vi "init_electron_count_Q.vi"(2 "max queue size (-1, unlimited)":i32) -> (8 "Electron Count Q Out":T1)   [LabVIEW 2023]
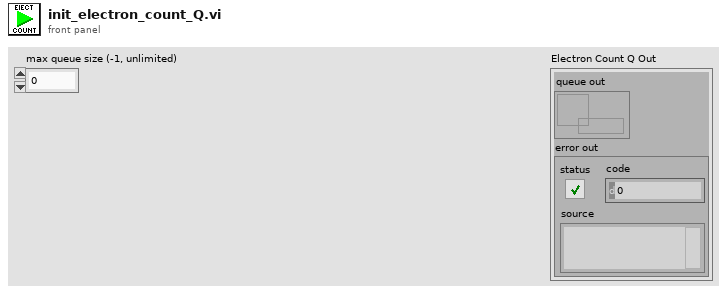
[diagram p1: front panel]
types:
  T1 = cluster{"queue out":refnum<queue>, "error out":errorcluster}
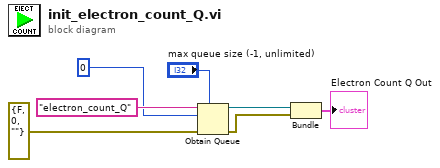
[diagram p0: block diagram]
diagram:
  n1 = Obtain Queue(max queue size (-1, unlimited)="max queue size (-1, unlimited)", name (unnamed)="electron_count_Q", element data type=0, error in (no error)=errorcluster {"status"=FALSE, "code"=0, "source"=""}) -> (queue out=w7:refnum<queue>, error out=w6:errorcluster)  [unwired: 1 in, 1 out]
  n2 = Bundle("queue out"=w7, "error out"=w6) -> (→"Electron Count Q Out":T1)  [unwired: 1 in]
